vi "Pulse Enable.vi"(8 "error in (no error)":errorcluster, 9 "Value":u8 format="%.0x", 10 "Session in":refnum<class "Session.lvclass">, 11 "PCF8574 I2C LCD in":refnum<class "PCF8574 I2C LCD.lvclass">) -> (0 "error out":errorcluster, 2 "Session out":refnum<class "Session.lvclass">, 3 "PCF8574 I2C LCD out":refnum<class "PCF8574 I2C LCD.lvclass">)   [LabVIEW 2020, in "CTI-Peripheral.lvlib" / "PCF8574 I2C LCD.lvclass"]
uses:
  PCF8574 I2C LCD.lvclass
  CTI/Session/Session.lvclass
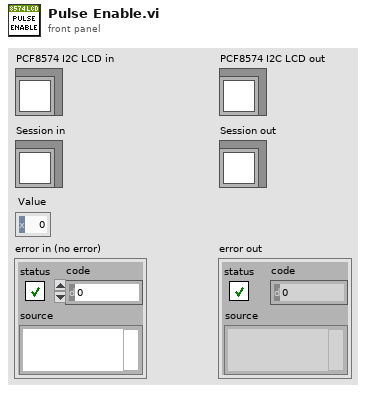
[diagram p1: front panel]
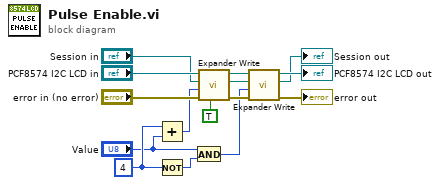
[diagram p0: block diagram]
diagram:
  w7 = u8 4
  n1 = Add(x=w7, y="Value") -> (x+y=w5:u8)
  n2 = Not(x=w7) -> (.not. x?=w6:u8)
  n3 = And(x="Value", y=w6) -> (x .and. y?=w3:u8)
  n4 = call "Expander Write.vi"("NoStop (F)"=TRUE, "error in (no error)"="error in (no error)", "Value"=w5, "Session in"="Session in", "PCF8574 I2C LCD in"="PCF8574 I2C LCD in") -> ("error out"=w14:errorcluster, "Session out"=w9:refnum<class "Session.lvclass">, "PCF8574 I2C LCD out"=w11:refnum<class "PCF8574 I2C LCD.lvclass">)  [unwired: 4 in]
  n5 = call "Expander Write.vi"("error in (no error)"=w14, "Value"=w3, "Session in"=w9, "PCF8574 I2C LCD in"=w11) -> ("error out"=→"error out":errorcluster, "Session out"=→"Session out":refnum<class "Session.lvclass">, "PCF8574 I2C LCD out"=→"PCF8574 I2C LCD out":refnum<class "PCF8574 I2C LCD.lvclass">)  [unwired: 5 in]
